vi "Command Translate Distance Field.vi"(2 "Input Robot System Funtions":T1, 3 "Cmd Parameter 1":dbl, 4 "Cmd Parameter 2":dbl, 5 "Startup":bool) -> (0 "Output Robot System Functions":T1, 1 "Completed":bool)   [LabVIEW 2014]
uses:
  Subsystems VIs/Robot Commands.ctl
  Command Execution State.ctl
  Global Variables/Sensor Data (Edited).vi
panel:
  # "Sample robot\ncontrol output.\nReplace with \nactual teleop \ncontrol signal \nstructure."
  # "Field Centric"
  # "Field Centric"
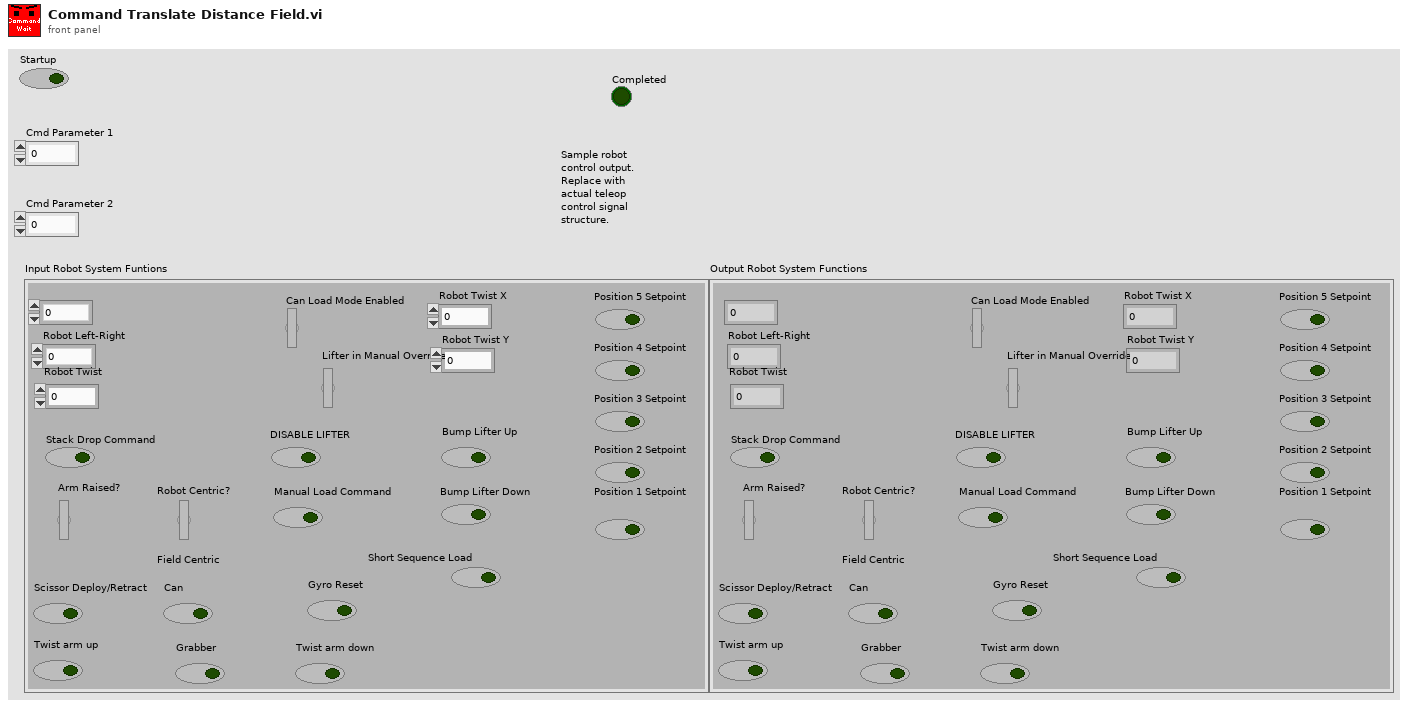
[diagram p1: front panel]
types:
  T1 = typedef "Robot Commands.ctl" = cluster{"Robot Forward-Reverse":dbl, "Robot Left-Right":dbl, "Robot Twist":dbl, "Can Load Mode Enabled":bool, "Lifter in Manual Override?":bool, "Stack Drop Command":bool, "Arm Raised?":bool, "DISABLE LIFTER":bool, "Position 1 Setpoint":bool, "Position 2 Setpoint":bool, "Position 3 Setpoint":bool, "Position 4 Setpoint":bool, "Position 5 Setpoint":bool, "Bump Lifter Down":bool, "Bump Lifter Up":bool, "Manual Load Command":bool, "Robot Centric?":bool, "Scissor Deploy/Retract":bool, "Grabber":bool, "Can":bool, "Twist arm up":bool, "Gyro Reset":bool, "Twist arm down":bool, "Short Sequence Load":bool, "Robot Twist X":dbl, "Robot Twist Y":dbl}
  T2 = typedef "Command Execution State.ctl" = enum16{"Initialize", "Execute", "Finish"}
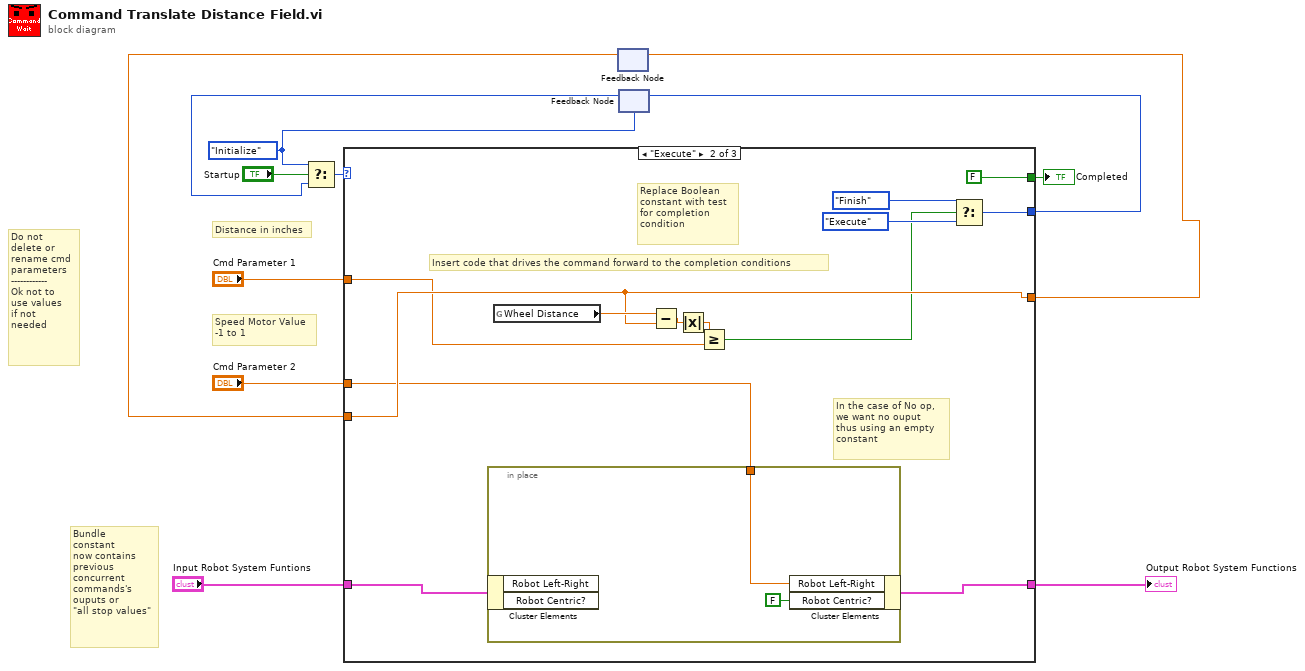
[diagram p0: block diagram]
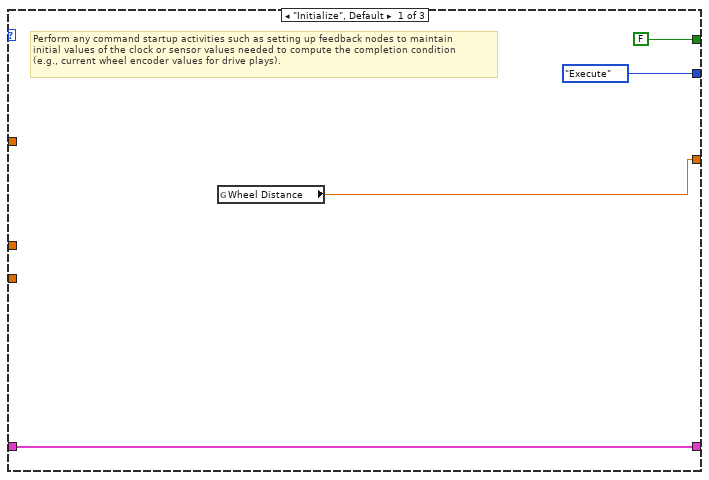
[diagram p2: hidden frame]
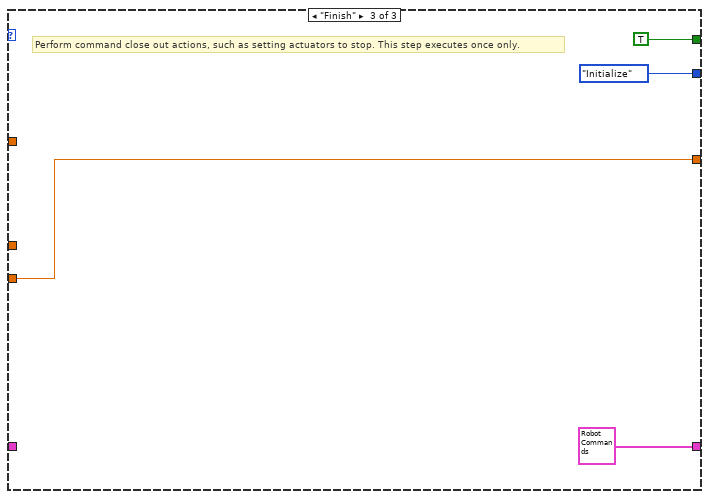
[diagram p3: hidden frame]
diagram:
  w7 = Command_Execution_State."Initialize" ("Play State")
  # "Bundle \nconstant\nnow contains\nprevious \nconcurrent\ncommands's\nouputs or\n\"all stop values\""
  # "Do not \ndelete or\nrename cmd\nparameters\n------------\nOk not to \nuse values\nif not \nneeded"
  # "Speed Motor Value\n-1 to 1"
  # "Distance in inches"
  n1 = feedback #1() -> (w1:dbl)  [unwired: 1 in]
  n2 = feedback #2(w7) -> (w8:T2)
  n3 = Select(t=w7, s="Startup", f=w8) -> (s? t:f=w12:T2)
  n4 = case shown="\"Execute\"" w12 {
    tunnel: [FALSE FALSE TRUE] -> w10
    tunnel: [Command_Execution_State."Execute" ("Play State") w22 Command_Execution_State."Initialize" ("f")] -> w9
    tunnel: "Cmd Parameter 1" -> [_ w19 _]
    tunnel: "Cmd Parameter 2" -> [_ w24 _]
    tunnel: [w14 w27 T1 {"Robot Forward-Reverse"=0.0, "Robot Left-Right"=0.0, "Robot Twist"=0.0, "Can Load Mode Enabled"=FALSE, "Lifter in Manual Override?"=FALSE, "Stack Drop Command"=FALSE, "Arm Raised?"=FALSE, "DISABLE LIFTER"=FALSE, "Position 1 Setpoint"=FALSE, "Position 2 Setpoint"=FALSE, "Position 3 Setpoint"=FALSE, "Position 4 Setpoint"=FALSE, "Position 5 Setpoint"=FALSE, "Bump Lifter Down"=FALSE, "Bump Lifter Up"=FALSE, "Manual Load Command"=FALSE, "Robot Centric?"=FALSE, "Scissor Deploy/Retract"=FALSE, "Grabber"=FALSE, "Can"=FALSE, "Twist arm up"=FALSE, "Gyro Reset"=FALSE, "Twist arm down"=FALSE, "Short Sequence Load"=FALSE, "Robot Twist X"=0.0, "Robot Twist Y"=0.0} ("Input Robot System Funtions")] -> w3
    tunnel: "Input Robot System Funtions" -> [w14 w28 _]
    tunnel: [w13 w25 w32] -> w2
    tunnel: w1 -> [_ w25 w32]
    frame "Initialize", Default {
      # "Perform any command startup activities such as setting up feedback nodes to maintain \ninitial values of the clock or sensor values needed to compute the completion condition\n(e.g., current wheel encoder values for drive plays)."
      n5 = global read "Sensor Data (Edited).vi" "Wheel Distance"() -> (w13:dbl)
    }
    frame "Execute" {
      # "In the case of No op, \nwe want no ouput \nthus using an empty \nconstant"
      # "Replace Boolean\nconstant with test \nfor completion \ncondition"
      # "Insert code that drives the command forward to the completion conditions"
      n6 = in-place {
        in-place-border: w24 -> [w31]
        n7 = in-place-cluster #3(w28) -> ()  [unwired: 2 out]
        n8 = in-place-cluster #3("Robot Left-Right"=w31, "Robot Centric?"=FALSE) -> (w27:T1)
      }
      n9 = global read "Sensor Data (Edited).vi" "Wheel Distance"() -> (w26:dbl)
      n10 = Subtract(x=w26, y=w25) -> (x-y=w18:dbl)
      n11 = Absolute Value(x=w18) -> (abs(x)=w17:dbl)
      n12 = Greater Or Equal?(x=w17, y=w19) -> (x >= y?=w21:bool)
      n13 = Select(t=Command_Execution_State."Finish" ("Play State"), s=w21, f=Command_Execution_State."Execute" ("Play State")) -> (s? t:f=w22:T2)
    }
    frame "Finish" {
      # "Perform command close out actions, such as setting actuators to stop. This step executes once only."
    }
  }
  "Completed" <- w10
  "Output Robot System Functions" <- w3
  n14 = feedback-in #1(w2) -> ()
  n15 = feedback-in #2(w9) -> ()
